vi "Player Bar Control.vi"(7 "IMAQ Image Display Ref":refnum<vi>) -> ()   [LabVIEW 2016]
uses:
  <vilib>/event_ctls.llb/lveventtype.ctl
  <vilib>/Utility/miscctls.llb/LVPointTypeDef.ctl
  User32.dll
panel:
  in  "Ctl Refnum":refnum<vi>
  out "Frame Indicator":cluster{"Current Frame":u16, "Total Frames":u16}
  in  "Step Forward":bool
  in  "Step Backwards":bool
  in  "Play":bool
  in  "Progress Bar":u16(slide) scale=0.0..100.0
  in  "Speed Selection":enum32{"Fast", "Medium", "Slow"}(radio)
  in  "Speed":bool
  # "/"
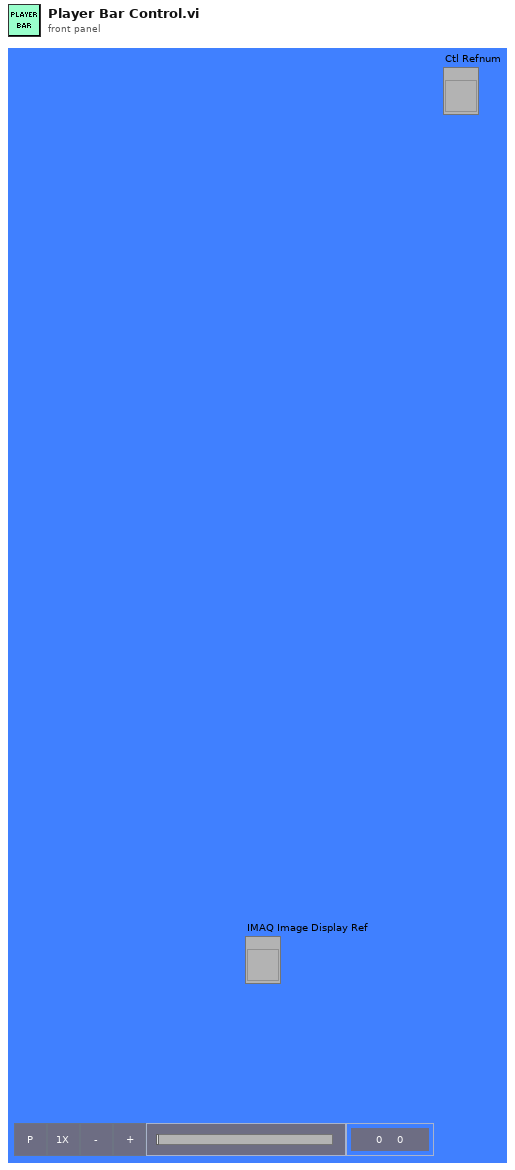
[diagram p1: front panel]
types:
  T1 = typedef "LVPointTypeDef.ctl" = cluster{"Horizontal":i16, "Vertical":i16}
  T2 = enum16{"Always On", "Always Off", "Off While Running"}
  T3 = enum32{"Invalid", "Standard", "Closed", "Hidden", "Minimized", "Maximized"}
  T4 = typedef "LVRectTypeDef.ctl" = cluster{"Left":i16, "Top":i16, "Right":i16, "Bottom":i16}
  T5 = typedef "lveventtype.ctl" = enum32{"Null", "Timeout", "Annotation Menu Selection", "Annotation Menu Selection?", "App Instance Close", "App Instance Close?", "Autoscale Range Change", "Bookmark Info Change", "Cell Edit", "Cell Edit?", "Cursor Grab", "Cursor Grab?", "Cursor Menu Selection", "Cursor Menu Selection?", "Cursor Move", "Cursor Release", "Data Change", "Direction Change", "Display State Change", "Drag Ended", "Drag Enter", "Drag Leave", "Drag Over", "Drag Source Update", "Drag Starting", "Drag Starting?", "Drop", "Exec State Change", "Key Down", "Key Down?", "Key Repeat", "Key Repeat?", "Key Up", "Listbox Double Click", "Menu Activation?", "Menu Selection (App)", "Menu Selection? (App)", "Menu Selection (User)", "Mouse Down", "Mouse Down?", "Mouse Enter", "Mouse Leave", "Mouse Move", "Mouse Up", "Mouse Wheel", "NI Security User Change (App)", "Pane Size", "Panel Close", "Panel Close?", "Panel Resize", "Plot Attribute Change", "Scale Range Change", "Shortcut Menu Activation?", "Shortcut Menu Selection (App)", "Shortcut Menu Selection? (App)", "Shortcut Menu Selection (User)", "Tree Double Click", "Tree Drag", "Tree Drag?", "Tree Drop", "Tree Drop?", "Tree Item Close", "Tree Item Close?", "Tree Item Open", "Tree Item Open?", "User Event", "Value Change"}
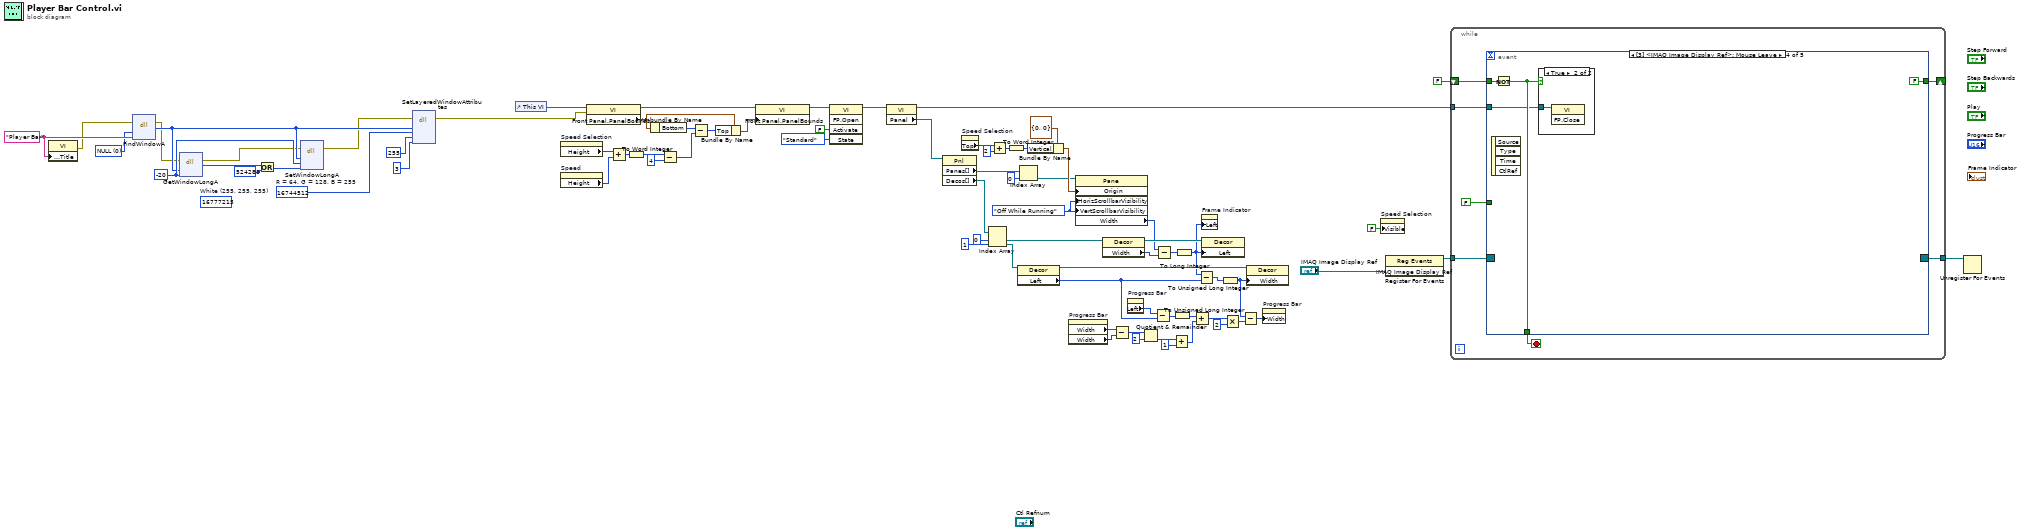
[diagram p0: block diagram]
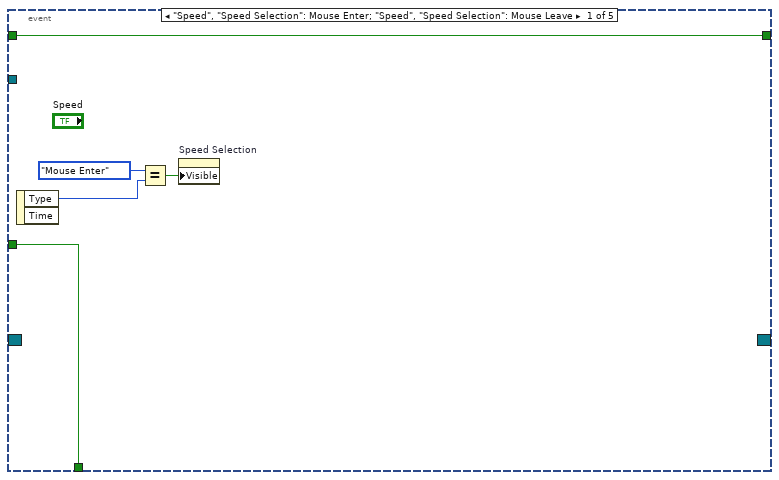
[diagram p2: hidden frame]
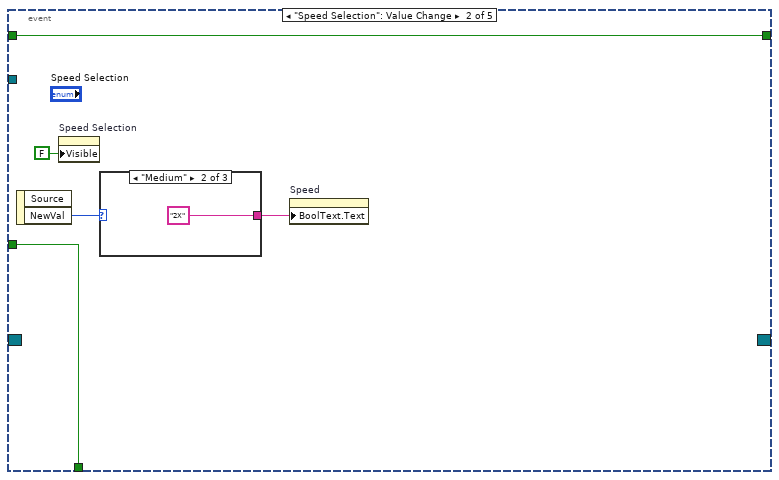
[diagram p3: hidden frame]
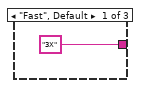
[diagram p4: hidden frame]
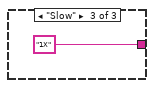
[diagram p5: hidden frame]
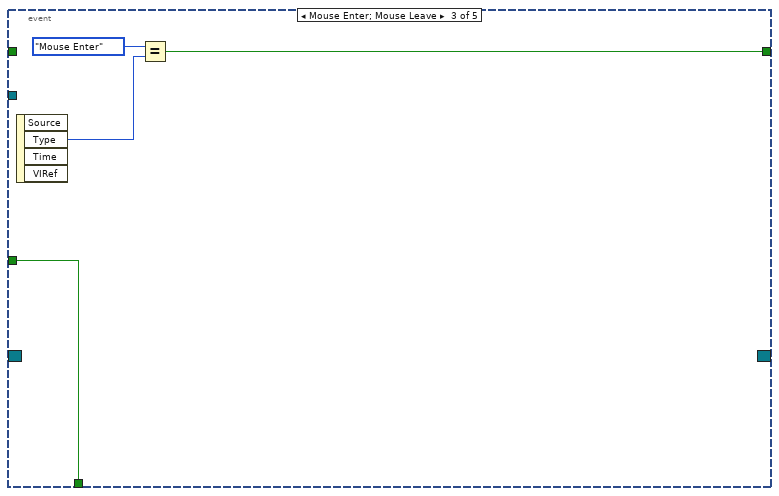
[diagram p6: hidden frame]
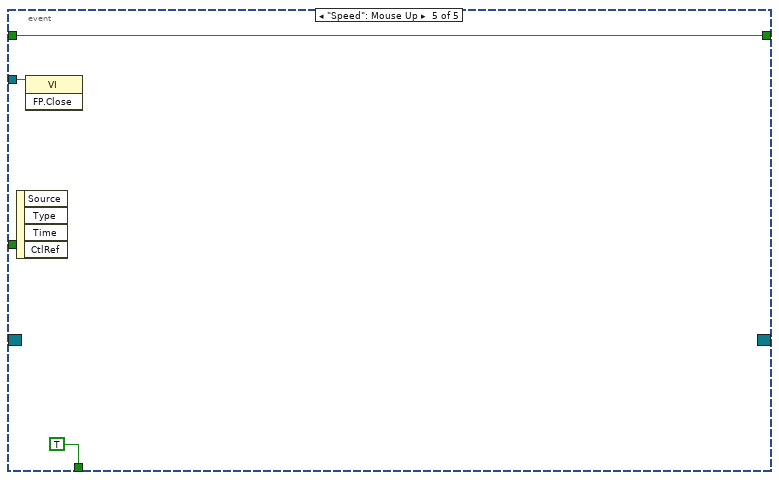
[diagram p8: hidden frame]
diagram:
  w32 = T2."Off While Running" ("Horizontal Scrollbar Visibility")
  w48 = 16744512  # R = 64, G = 128, B = 255
  (unwired) 16777215  # White (255, 255, 255)
  w54 = 0 items=["NULL"]
  w58 = -20 ("nIndex")
  w60 = "Player Bar" ("Front Panel Window:Title")
  n1 = property class="VI"("Front Panel.Title"=w60) -> (error out=w47:errorcluster)  [unwired: 2 in, 1 out]
  n2 = dll-call lib="user32.dll" fn="FindWindowA" label="FindWindow"(error in=w47, "lpszClassName"=w54, "lpszWindowName"=w60) -> (error out=w51:errorcluster, "hWnd"=w57:i32)  [unwired: 3 in, 2 out]
  n3 = dll-call lib="USER32.DLL" fn="GetWindowLongA" label="getWindowLong"(error in=w51, "handle"=w57, "nIndex"=w58) -> (error out=w50:errorcluster, w56:i32)  [unwired: 4 in, 1 out]
  n4 = Or(x=w56, y=524288) -> (x .or. y?=w59:i32)
  n5 = dll-call lib="USER32.DLL" fn="SetWindowLongA" label="SetWindowLong"(error in=w50, "handle"=w57, "nIndex"=w58, "dwNewLong"=w59) -> (error out=w49:errorcluster)  [unwired: 5 in, 2 out]
  n6 = dll-call lib="USER32.DLL" fn="SetLayeredWindowAttributes" label="SetLayeredWindowAttributs"(error in=w49, "handle"=w57, "crkey"=w48, "bAlpha"=255, "dwFlags"=3) -> (error out=w46:errorcluster)  [unwired: 6 in, 2 out]
  n7 = control-ref of="This VI"() -> (w76:refnum<vi>)
  n8 = property on="Speed Selection" class="RadioBtnsControl (strict)"() -> ("Height"=w70:u32)  [unwired: 2 in, 2 out]
  n9 = property on="Speed" class="Bool (strict)"() -> ("Height"=w71:u32)  [unwired: 2 in, 2 out]
  n10 = property class="VI"(reference=w76, error in=w46) -> (reference out=w67:refnum<vi>, "Front Panel.PanelBounds"=w66:T4)  [unwired: 1 out]
  n11 = Add(x=w70, y=w71) -> (x+y=w65:u32)
  n12 = To Word Integer(number=w65) -> (16bit integer=w62:i16)
  n13 = Unbundle By Name(w66) -> ("Bottom"=w68:i16)
  n14 = Subtract(x=w62, y=i16 4) -> (x-y=w63:i16)
  n15 = Subtract(x=w68, y=w63) -> (x-y=w61:i16)
  n16 = Bundle By Name(cluster=w66, "Top"=w61) -> (w69:T4)
  n17 = property class="VI"(reference=w67, "Front Panel.PanelBounds"=w69) -> (reference out=w43:refnum<vi>)  [unwired: 1 in, 1 out]
  n18 = invoke class="VI" method="FP.Open"(reference=w43, "Activate"=FALSE ("Activate?"), "State"=T3."Standard") -> (reference out=w3:refnum<vi>)  [unwired: 2 in, 4 out]
  n19 = property class="VI"(reference=w3) -> (reference out=w2:refnum<vi>, "Panel"=w42:refnum<vi>)  [unwired: 1 in, 1 out]
  n20 = property class="Pnl"(reference=w42) -> ("Panes[]"=w35:refnum<vi>[], "Decos[]"=w31:refnum<vi>[])  [unwired: 1 in, 2 out]
  n21 = property on="Speed Selection" class="RadioBtnsControl (strict)"() -> ("Top"=w39:i32)  [unwired: 2 in, 2 out]
  n22 = Index Array(array=w31, index #1=0 ("index"), index #2=1 ("index")) -> (element #1=w29:refnum<vi>, element #2=w23:refnum<vi>)
  n23 = Add(x=w39, y=2) -> (x+y=w40:i32)
  n24 = To Word Integer(number=w40) -> (16bit integer=w41:i16)
  n25 = property class="Decor"(reference=w23) -> (reference out=w22:refnum<vi>, "Left"=w21:i32)  [unwired: 1 in, 1 out]
  n26 = Index Array(array=w35, index=0) -> (element=w33:refnum<vi>)
  n27 = Bundle By Name(cluster=T1 {"Horizontal"=0, "Vertical"=0} ("Origin"), "Vertical"=w41) -> (w37:T1)
  n28 = property on="Progress Bar" class="Slide (strict)"() -> ("Width"=w17:u32, "Width"=w16:u32)  [unwired: 2 in, 2 out]
  n29 = property class="Pane"(reference=w33, "Origin"=w37, "HorizScrollbarVisibility"=w32, "VertScrollbarVisibility"=w32) -> ("Width"=w25:u32)  [unwired: 1 in, 2 out]
  n30 = property class="Decor"(reference=w29) -> (reference out=w28:refnum<vi>, "Width"=w26:u32)  [unwired: 1 in, 1 out]
  n31 = Subtract(x=w17, y=w16) -> (x-y=w13:u32)
  n32 = property on="Progress Bar" class="Slide (strict)"() -> ("Left"=w20:i32)  [unwired: 2 in, 2 out]
  n33 = Quotient & Remainder(x=w13, y=u32 2) -> (floor(x/y)=w9:u32)  [unwired: 1 out]
  n34 = Subtract(x=w20, y=w21) -> (x-y=w11:i32)
  n35 = Subtract(x=w25, y=w26) -> (x-y=w27:u32)
  n36 = To Unsigned Long Integer(number=w11) -> (unsigned 32bit integer=w4:u32)
  n37 = Add(x=w9, y=u32 1) -> (x+y=w7:u32)
  n38 = To Long Integer(number=w27) -> (32bit integer=w19:i32)
  n39 = Add(x=w4, y=w7) -> (x+y=w10:u32)
  n40 = Subtract(x=w19, y=w21) -> (x-y=w18:i32)
  n41 = property on="Frame Indicator" class="Clust (strict)"("Left"=w19) -> ()  [unwired: 2 in, 2 out]
  n42 = property class="Decor"(reference=w28, "Left"=w19) -> ()  [unwired: 1 in, 2 out]
  n43 = To Unsigned Long Integer(number=w18) -> (unsigned 32bit integer=w6:u32)
  n44 = Multiply(x=w10, y=u32 2) -> (x*y=w14:u32)
  n45 = Subtract(x=w6, y=w14) -> (x-y=w5:u32)
  n46 = property class="Decor"(reference=w22, "Width"=w6) -> ()  [unwired: 1 in, 2 out]
  n47 = property on="Progress Bar" class="Slide (strict)"("Width"=w5) -> ()  [unwired: 2 in, 2 out]
  n48 = property on="Speed Selection" class="RadioBtnsControl (strict)"("Visible"=FALSE) -> ()  [unwired: 2 in, 2 out]
  n49 = register-events("IMAQ Image Display Ref") -> (reference out=w73:refnum<event-registration>)  [unwired: 2 in, 1 out]
  n50 = while {
    tunnel: w2 -> [w81]
    shift-right: [w80] -> _
    shift-left: FALSE -> [w79]
    tunnel: w73 -> [w78]
    tunnel: [w77] -> w72
    stop <- w82 stop-if-true
    n51 = event shown="[3] <IMAQ Image Display Ref>: Mouse Leave" {
      selector: w78 -> [_ _ _ _ _]
      dyn-events: [_ _ _ _ _] -> w77
      timeout: _ -> [_ _ _ _ _]
      tunnel: FALSE -> [w85 w92 w100 _ _]
      tunnel: [w85 w92 w100 w103 TRUE] -> w82
      tunnel: w81 -> [_ _ _ w101 w108]
      tunnel: [w84 w91 w97 FALSE w106] -> w80
      tunnel: w79 -> [w84 w91 _ w104 w106]
      event "Speed", "Speed Selection": Mouse Enter; "Speed", "Speed Selection": Mouse Leave {
        n52 = event-data() -> ("Type"=w87:T5)  [unwired: 1 in, 1 out]
        n53 = Equal?(x=lveventtype."Mouse Enter" ("Type"), y=w87) -> (x = y?=w86:bool)
        n54 = property on="Speed Selection" class="RadioBtnsControl (strict)"("Visible"=w86) -> ()  [unwired: 2 in, 2 out]
      }
      event "Speed Selection": Value Change {
        n55 = event-data() -> ("NewVal"=w90:enum32{"Fast", "Medium", "Slow"})  [unwired: 1 in, 1 out]
        n56 = property on="Speed Selection" class="RadioBtnsControl (strict)"("Visible"=FALSE) -> ()  [unwired: 2 in, 2 out]
        n57 = case shown="\"Medium\"" w90 {
          tunnel: ["3X" "2X" "1X"] -> w89
          frame "Fast", Default {
          }
          frame "Medium" {
          }
          frame "Slow" {
          }
        }
        n58 = property on="Speed" class="Bool (strict)"("BoolText.Text"=w89) -> ()  [unwired: 2 in, 2 out]
      }
      event Mouse Enter; Mouse Leave {
        n59 = event-data() -> ("Type"=w99:T5)  [unwired: 1 in, 3 out]
        n60 = Equal?(x=lveventtype."Mouse Enter" ("Type"), y=w99) -> (x = y?=w97:bool)
      }
      event Mouse Leave {
        n61 = event-data() -> ()  [unwired: 1 in, 4 out]
        n62 = Not(x=w104) -> (.not. x?=w103:bool)
        n63 = case shown="True" w103 {
          tunnel: w101 -> [_ w105]
          frame False {
          }
          frame True {
            n64 = invoke class="VI" method="FP.Close"(reference=w105) -> ()  [unwired: 2 in, 3 out]
          }
        }
      }
      event "Speed": Mouse Up {
        n65 = event-data() -> ()  [unwired: 1 in, 4 out]
        n66 = invoke class="VI" method="FP.Close"(reference=w108) -> ()  [unwired: 2 in, 3 out]
      }
    }
  }
  n67 = Unregister For Events(event registration refnum=w72) -> ()  [unwired: 1 in, 1 out]
